vi "多电机同时初始化.vi"(8 "error in (no error)":errorcluster caption="错误输入（无错误）") -> (0 "error out":errorcluster caption="错误输出")   [LabVIEW 2017]
doc: "该模板用于创建子VI。"
panel:
  out "Position 5":dbl[](array[numeric]) format="%.6f"
  out "error out 2":errorcluster
  out "Position 4":dbl[](array[numeric]) format="%.6f"
  out "Position 3":dbl[](array[numeric]) format="%.6f"
  out "Identification 2":string
  out "SN out 2":string
  out "Position 2":dbl[](array[numeric]) format="%.6f"
  out "Device ID out 2":i32
  out "Identification":string
  out "SN out":string
  out "Device ID out":i32
  out "Position":dbl[](array[numeric]) format="%.6f"
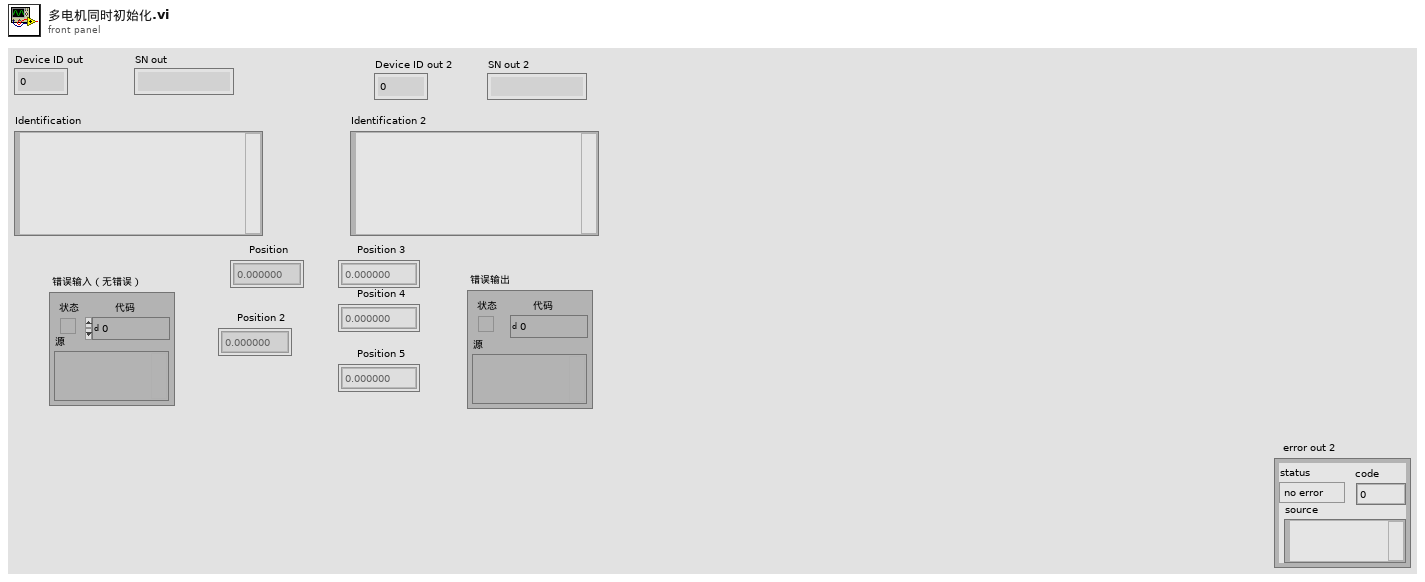
[diagram p1: front panel]
types:
  T1 = cluster{"Register DC":bool, "DaisyChain Search?":bool, "Device ID":i32}
  T2 = cluster{"RON Affected axes":string[], "Reference mode":bool[], "Check FRF?":bool}
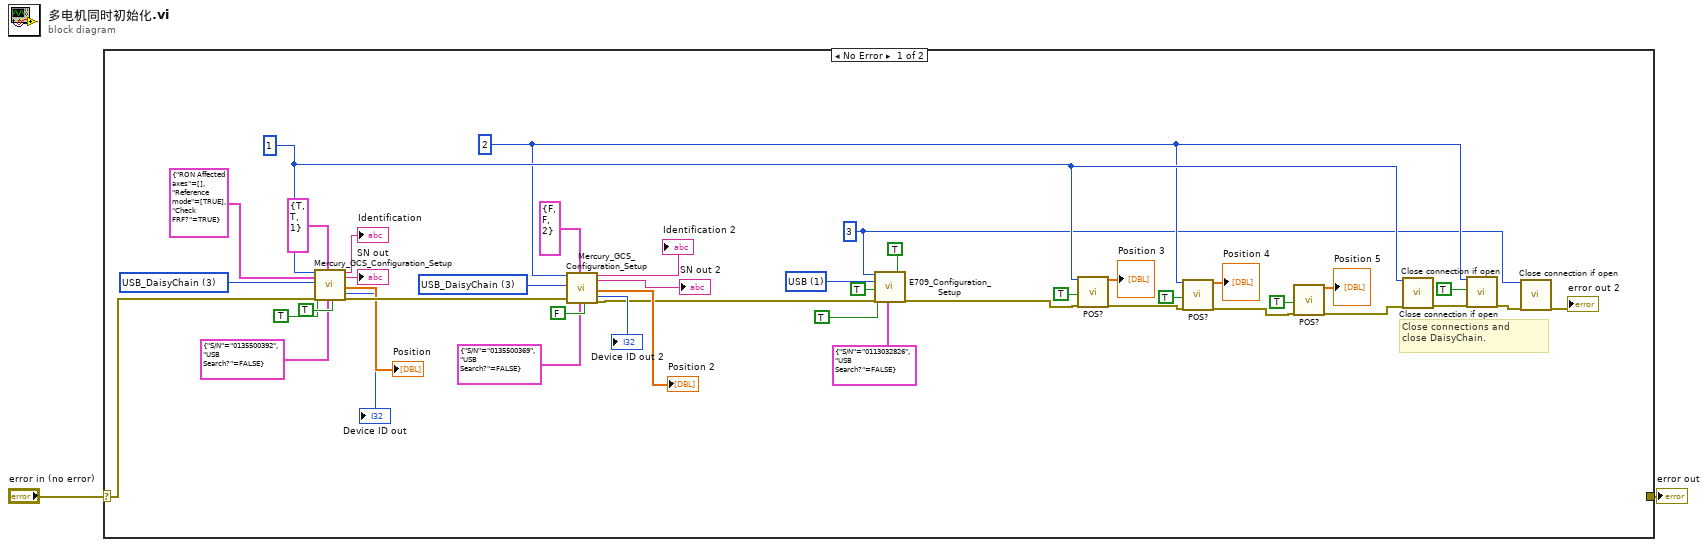
[diagram p0: block diagram]
diagram:
  n1 = case shown="No Error" "error in (no error)" {
    selector: "error in (no error)" -> [w44 w46]
    tunnel: [_ w46] -> w1
    frame No Error {
      w13 = u16 1 items=["RS232", "USB"] ("Interface")
      w3 = 3 ("System no.")
      w32 = u16 3 items=["RS232", "RS232 DaisyChain", "USB", "USB_DaisyChain"] ("Interface")
      w45 = u16 3 items=["RS232", "RS232 DaisyChain", "USB", "USB_DaisyChain"] ("Interface")
      w17 = 2 ("System no.")
      w18 = 1 ("System no.")
      # "Close connections and\nclose DaisyChain."
      n2 = call "Mercury_GCS_Configuration_Setup.vi"("System no."=w18, "RON settings"=T2 {"RON Affected axes"=[], "Reference mode"=[TRUE], "Check FRF?"=TRUE}, "Interface"=w45, "All axes?"=TRUE, "error in"=w44, "DaisyChain settings"=T1 {"Register DC"=TRUE, "DaisyChain Search?"=TRUE, "Device ID"=1}, "USB settings"=cluster{"S/N":string, "USB Search?":bool} {"S/N"="0135500392", "USB Search?"=FALSE}, "Switch servo on?"=TRUE) -> ("Device ID out"=→"Device ID out":i32, "Identification"=→"Identification":string, "SN out"=→"SN out":string, "Position"=→"Position":dbl[], "error out"=w38:errorcluster)  [unwired: 5 in, 2 out]
      n3 = call "Mercury_GCS_Configuration_Setup.vi"("System no."=w17, "Interface"=w32, "error in"=w38, "DaisyChain settings"=T1 {"Register DC"=FALSE, "DaisyChain Search?"=FALSE, "Device ID"=2}, "USB settings"=cluster{"S/N":string, "USB Search?":bool} {"S/N"="0135500369", "USB Search?"=FALSE}, "Switch servo on?"=FALSE) -> ("Device ID out"=→"Device ID out 2":i32, "Identification"=→"Identification 2":string, "SN out"=→"SN out 2":string, "Position"=→"Position 2":dbl[], "error out"=w16:errorcluster)  [unwired: 7 in, 2 out]
      n4 = call "E709_Configuration_Setup.vi"("System no."=w3, "Interface"=w13, "Change servo status to ON?"=TRUE, "Perform autozero?"=TRUE, "error in"=w16, "USB settings"=cluster{"S/N":string, "USB Search?":bool} {"S/N"="0113032826", "USB Search?"=FALSE}, "Move to middle?"=TRUE) -> ("error out"=w10:errorcluster)  [unwired: 7 in, 5 out]
      n5 = call "POS?.vi"("System no."=w18, "All axes?"=TRUE, "error in"=w10) -> ("Position"=→"Position 3":dbl[], "error out"=w25:errorcluster)  [unwired: 15 in]
      n6 = call "POS?.vi"("System no."=w17, "All axes?"=TRUE, "error in"=w25) -> ("Position"=→"Position 4":dbl[], "error out"=w7:errorcluster)  [unwired: 15 in]
      n7 = call "POS?.vi"("All axes?"=TRUE, "error in"=w7) -> ("Position"=→"Position 5":dbl[], "error out"=w6:errorcluster)  [unwired: 16 in]
      n8 = call "Close connection if open.vi"("System no."=w18, "error in"=w6) -> ("error out"=w20:errorcluster)  [unwired: 16 in, 1 out]
      n9 = call "Close connection if open.vi"("System no."=w17, "Close DaisyChain"=TRUE, "error in"=w20) -> ("error out"=w5:errorcluster)  [unwired: 15 in, 1 out]
      n10 = call "Close connection if open.vi"("System no."=w3, "error in"=w5) -> ("error out"=→"error out 2":errorcluster)  [unwired: 16 in, 1 out]
    }
    frame Error {
    }
  }
  "error out" <- w1
